vi "Update Header Colours.vi"(8 "error in (no error)":errorcluster, 11 "Hex Viewer in":refnum<class "Hex Viewer.lvclass">) -> (0 "error out":errorcluster)   [LabVIEW 2021, in "Hex Viewer.lvclass"]
uses:
  Hex Viewer.lvclass
  <vilib>/Utility/miscctls.llb/LVRowAndColumnTypeDef.ctl
  Hex Viewer.lvclass/Hex Viewer.ctl
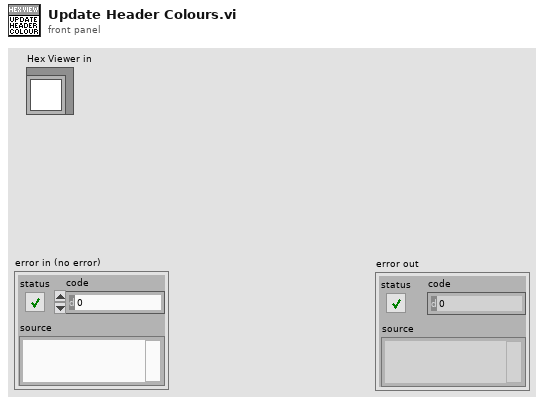
[diagram p1: front panel]
types:
  T1 = typedef "LVRowAndColumnTypeDef.ctl" = cluster{"Row":i32, "Column":i32}
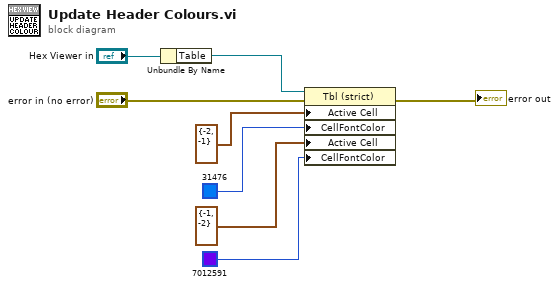
[diagram p0: block diagram]
diagram:
  n1 = Unbundle By Name("Hex Viewer in") -> ("Table"=w3:refnum<vi>)
  n2 = property class="Tbl (strict)"(reference=w3, error in="error in (no error)", "Active Cell"=T1 {"Row"=-2, "Column"=-1} ("Active Cell:Active Cell"), "CellFontColor"=u32 31476, "Active Cell"=T1 {"Row"=-1, "Column"=-2} ("Active Cell:Active Cell"), "CellFontColor"=u32 7012591) -> (error out=→"error out":errorcluster)  [unwired: 1 out]
